vi "gearedMotorVelControl (SubVI).vi"(6 "Reset":bool, 8 "error in (no error)":errorcluster, 9 "PID gains":T1={"proportional gain (Kc)"=2.0, "integral time (Ti, min)"=0.01, "derivative time (Td, min)"=0.00010000000000000003}, 10 "Speed (degs)":dbl, 11 "dt":i64) -> (0 "error out":errorcluster, 1 "Waveform Chart":T2(graph), 2 "MotorEncoder (deg)":dbl)   [LabVIEW 2019, in "SJCube_ElvisIII.lvlib"]
uses:
  SJCube_ElvisIII.lvlib
  <vilib>/addons/control/pid/pid.llb/PID (DBL).vi
  <vilib>/addons/control/pid/NI_PID_pid.lvlib
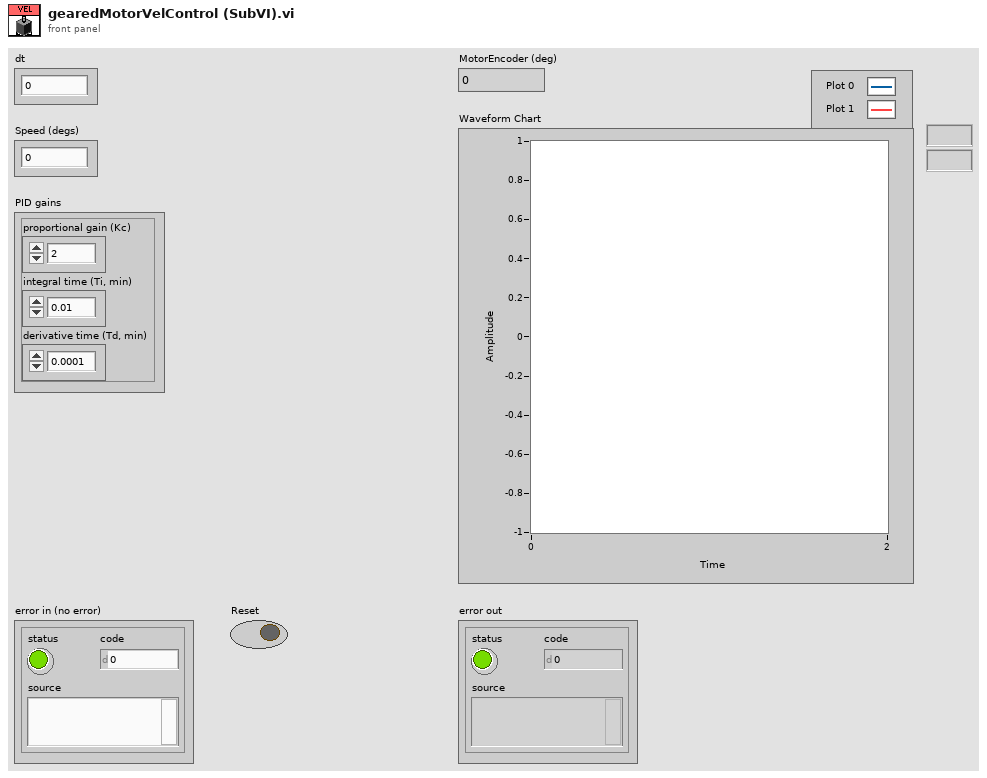
[diagram p1: front panel]
types:
  T1 = cluster{"proportional gain (Kc)":dbl, "integral time (Ti, min)":dbl, "derivative time (Td, min)":dbl}
  T2 = cluster{"Position (deg)":dbl, "MotorEncoder (deg)":dbl}
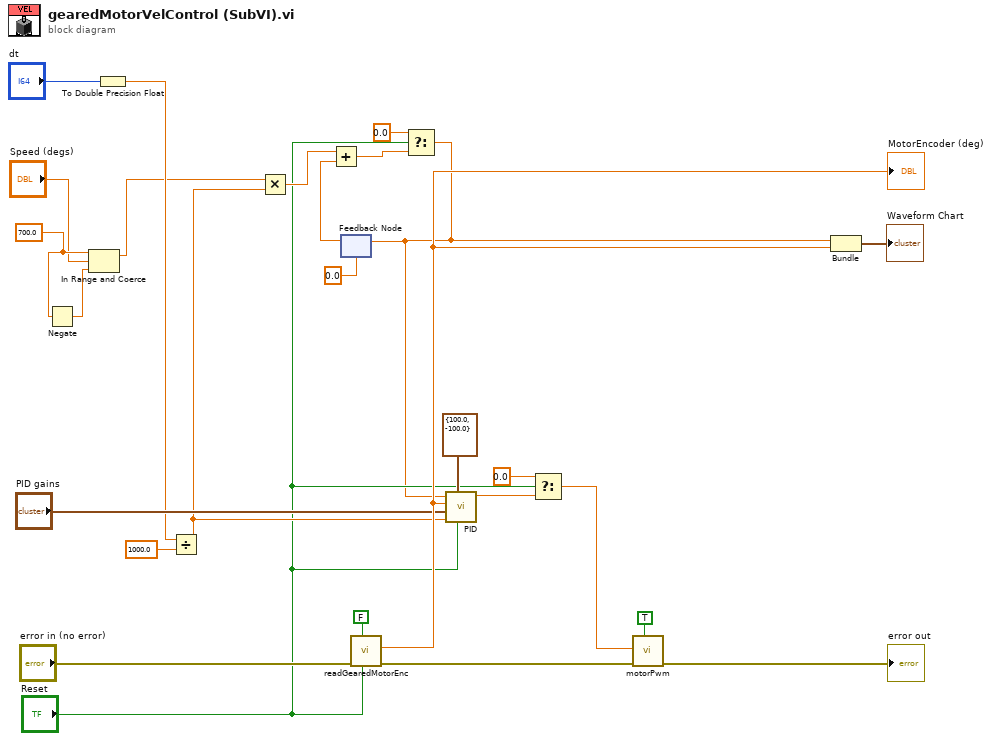
[diagram p0: block diagram]
diagram:
  w4 = 700.0 ("upper limit")
  n1 = Negate(x=w4) -> (-x=w3:dbl)
  n2 = In Range and Coerce(upper limit=w4, x="Speed (degs)", lower limit=w3) -> (coerced(x)=w1:dbl)  [unwired: 1 out]
  n3 = To Double Precision Float(number="dt") -> (double precision float=w14:dbl)
  n4 = Divide(x=w14, y=1000.0) -> (x/y=w12:dbl)
  n5 = Multiply(x=w1, y=w12) -> (x*y=w11:dbl)
  n6 = feedback #1(0.0) -> (w10:dbl)
  n7 = Add(x=w11, y=w10) -> (x+y=w6:dbl)
  n8 = call "readGearedMotorEnc.vi"("Reset Counter"="Reset", "Reverse ENC?"=FALSE, "error in (no error)"="error in (no error)") -> ("error out"=w20:errorcluster, "gearedMotorEncoder (deg)"=w25:dbl)  [unwired: 7 in]
  "MotorEncoder (deg)" <- w25
  n9 = Select(t=0.0, s="Reset", f=w6) -> (s? t:f=w5:dbl)
  n10 = feedback-in #1(w5) -> ()
  n11 = call-poly <vilib>:"PID.vi"("reinitialize? (F)"="Reset", "output range"=cluster{"output high":dbl, "output low":dbl} {"output high"=100.0, "output low"=-100.0}, "dt (s)"=w12, "PID gains"="PID gains", "process variable"=w25, "setpoint"=w5) -> ("output"=w23:dbl)  [unwired: 4 in, 1 out]
  n12 = Select(t=0.0, s="Reset", f=w23) -> (s? t:f=w24:dbl)
  n13 = call "motorPwm.vi"("reverse?"=TRUE, "error in (no error)"=w20, "Speed (PWM)"=w24) -> ("error out"=→"error out":errorcluster)  [unwired: 8 in]
  n14 = Bundle("t"=w5, "gearedMotorEncoder (deg)"=w25) -> (→"Waveform Chart":cluster{"t":dbl, "gearedMotorEncoder (deg)":dbl})  [unwired: 1 in]
